vi "TriggerTest.vi"() -> ()   [LabVIEW 2017]
panel:
  out "Number of multipliers":dbl
  in  "Stimulus Multipliers":string
  out "Current multiplier":dbl
  out "Current stimulus file":string
  out "Number of files Remaining":dbl
  out "Number of all files":dbl
  in  "Stimulus folder":path
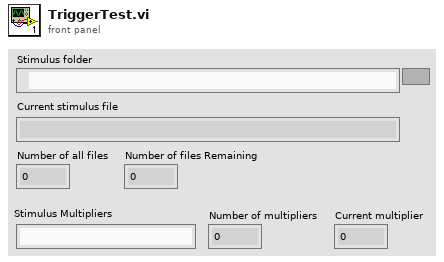
[diagram p1: front panel]
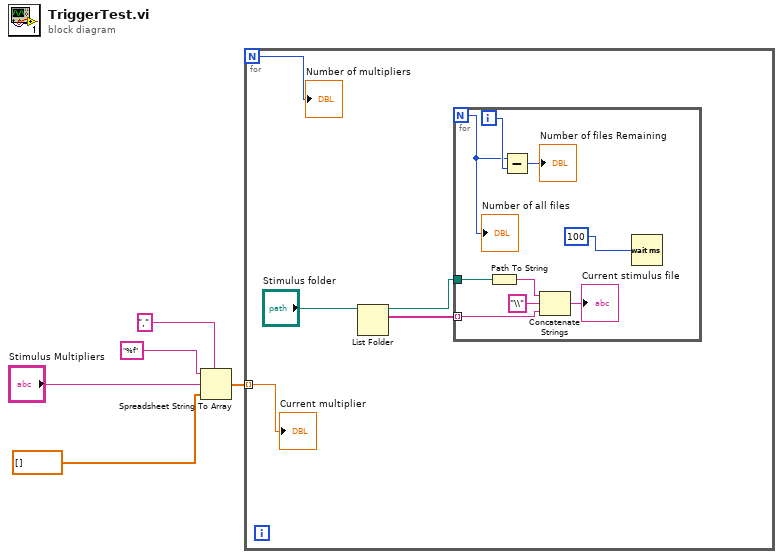
[diagram p0: block diagram]
diagram:
  n1 = Spreadsheet String To Array(delimiter (Tab)=",", format string="%f", spreadsheet string="Stimulus Multipliers", array type (2D Dbl)=dbl[] []) -> (array=w1:dbl[])
  n2 = for {
    N -> [w6]
    tunnel: w1 -> [w10] mode=indexing
    n3 = List Folder(path="Stimulus folder") -> (path out=w9:path, filenames=w8:string[])  [unwired: 3 in, 2 out]
    n4 = for {
      N -> [w12]
      tunnel: w8 -> [w15] mode=indexing
      tunnel: w9 -> [w19]
      i -> [w14]
      n5 = Path To String(path=w19) -> (string=w18:string)
      n6 = Subtract(x=w12, y=w14) -> (x-y=→"Number of files Remaining":i32)
      n7 = Concatenate Strings(w18, "\\", w15) -> (→"Current stimulus file":string)
      n8 = Wait (ms)(milliseconds to wait=100) -> ()  [unwired: 1 out]
      "Number of all files" <- w12
    }
    "Current multiplier" <- w10
    "Number of multipliers" <- w6
  }
